vi "adam-analog-data-read.vi"(8 "error in (no error)":errorcluster, 9 "overwrite-command":string, 10 "current-buffer":string, 11 "VISA Refnum in":refnum<visa-resource-name>) -> (0 "error out":errorcluster, 1 "return count":u32, 2 "read buffer":string, 3 "VISA Refnum Out":refnum<visa-resource-name>, 5 "Bytes at Port":u32)   [LabVIEW 2024]
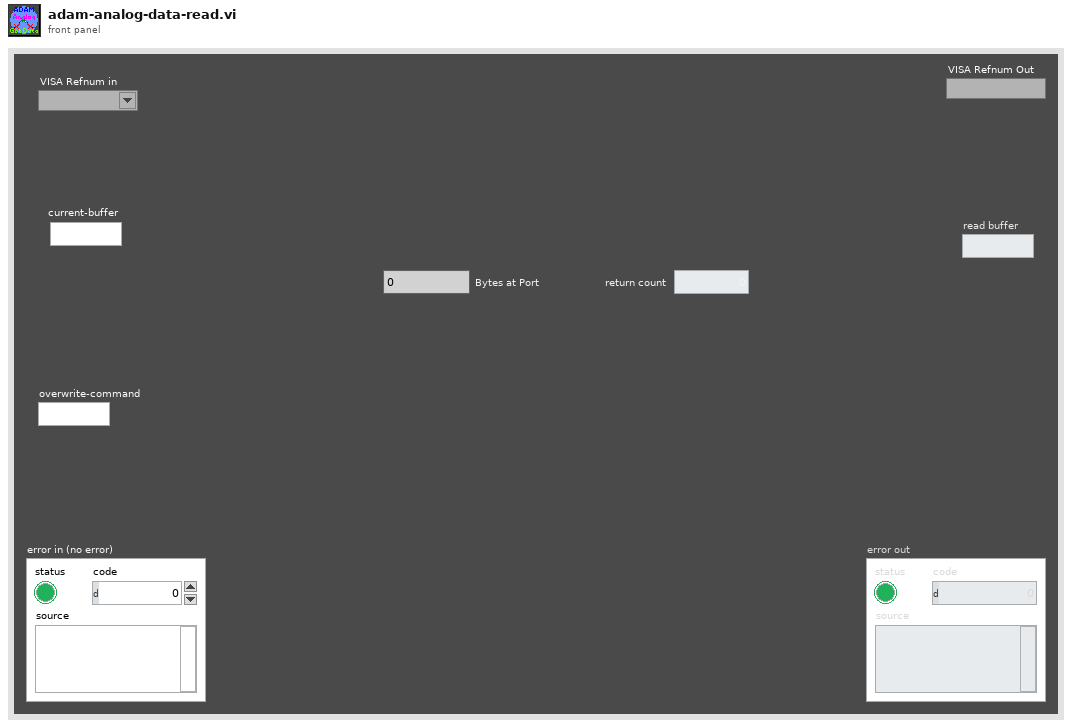
[diagram p1: front panel]
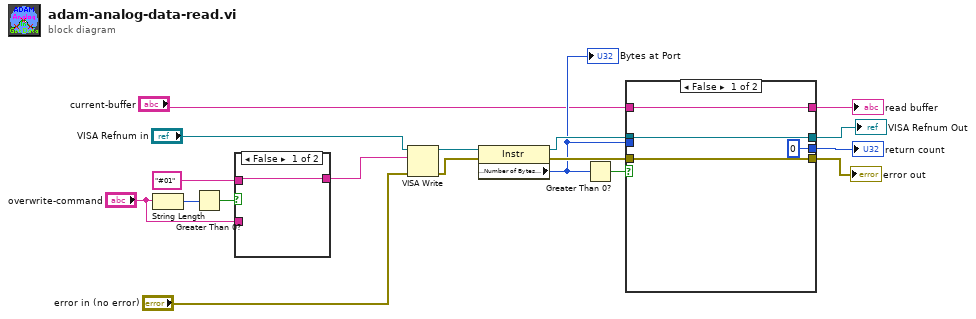
[diagram p0: block diagram]
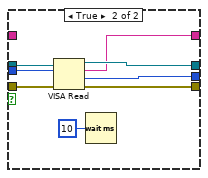
[diagram p3: hidden frame]
diagram:
  n1 = String Length(string="overwrite-command") -> (length=w13:i32)
  n2 = Greater Than 0?(x=w13) -> (x > 0?=w12:bool)
  n3 = case shown="False" w12 {
    tunnel: "overwrite-command" -> [_ w20]
    tunnel: "#01" ("write buffer") -> [w19 _]
    tunnel: [w19 w20] -> w9
    frame False {
    }
    frame True {
    }
  }
  n4 = VISA Write(VISA resource name="VISA Refnum in", write buffer=w9, error in (no error)="error in (no error)") -> (VISA resource name out=w15:refnum<visa-resource-name>, error out=w17:errorcluster)  [unwired: 1 out]
  n5 = property class="Instr"(reference=w15, error in=w17) -> (reference out=w8:refnum<visa-resource-name>, error out=w7:errorcluster, "Serial Settings:Number of Bytes at Serial Port"=w5:u32)
  "Bytes at Port" <- w5
  n6 = Greater Than 0?(x=w5) -> (x > 0?=w18:bool)
  n7 = case shown="False" w18 {
    tunnel: w7 -> [w23 w31]
    tunnel: w8 -> [w24 w32]
    tunnel: [w24 w30] -> w3
    tunnel: [w23 w29] -> w6
    tunnel: [w22 w28] -> w4
    tunnel: w5 -> [_ w26]
    tunnel: "current-buffer" -> [w22 _]
    tunnel: [u32 0 ("return count") w25] -> w1
    frame False {
    }
    frame True {
      n8 = VISA Read(VISA resource name=w32, byte count=w26, error in (no error)=w31) -> (VISA resource name out=w30:refnum<visa-resource-name>, read buffer=w28:string, return count=w25:u32, error out=w29:errorcluster)
      n9 = Wait (ms)(milliseconds to wait=u32 10) -> ()  [unwired: 1 out]
    }
  }
  "error out" <- w6
  "read buffer" <- w4
  "VISA Refnum Out" <- w3
  "return count" <- w1
